vi "Get SMO PGSQL Log Paths.vi"(8 "error in (no error)":errorcluster, 11 "instrument.Cryostation in":refnum<class "instrument.Cryostation.lvclass">) -> (0 "error out":errorcluster, 2 "Paths":string, 3 "instrument.Cryostation out":refnum<class "instrument.Cryostation.lvclass">)   [LabVIEW 2016, in "instrument.Cryostation.lvclass"]
uses:
  instrument.Cryostation.lvclass
  <userlib>/LevyLab/Levylab Instruments/Instrument Types/Cryostat/Instrument.Cryostat.lvclass
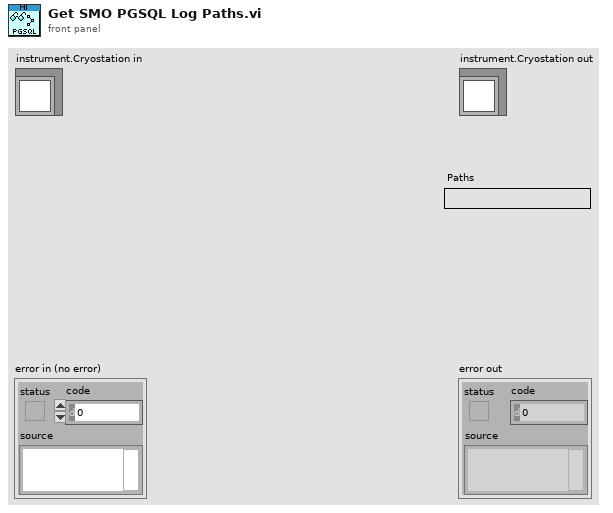
[diagram p1: front panel]
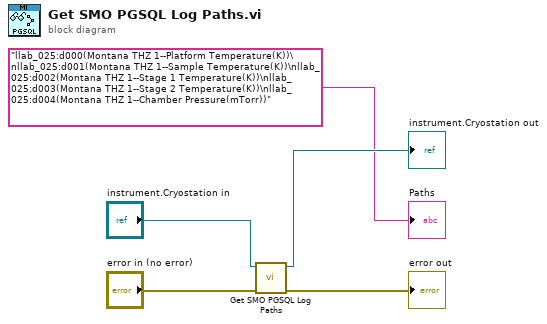
[diagram p0: block diagram]
diagram:
  n1 = call-parent "Get SMO PGSQL Log Paths.vi"("error in (no error)"="error in (no error)", "Instrument in"="instrument.Cryostation in") -> ("error out"=→"error out":errorcluster, "Instrument out"=→"instrument.Cryostation out":refnum<class "instrument.Cryostation.lvclass">)  [unwired: 7 in, 1 out]
  "Paths" <- "llab_025:d000(Montana THZ 1--Platform Temperature(K))\nllab_025:d001(Montana THZ 1--Sample Temperature(K))\nllab_025:d002(Montana THZ 1--Stage 1 Temperature(K))\nllab_025:d003(Montana THZ 1--Stage 2 Temperature(K))\nllab_025:d004(Montana THZ 1--Chamber Pressure(mTorr))" ("Paths")
